vi "TurnToAngle-C.vi"(11 "Params":string[][](array[string])) -> ()   [LabVIEW 2017]
uses:
  C:/Users/Bendethic/Documents/LabVIEW Data/Projects/2018 Power Up/FRC_PracticeBot-2018/Robot Project/Framework/Robot Global Data.vi
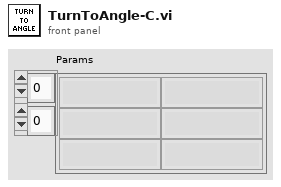
[diagram p1: front panel]
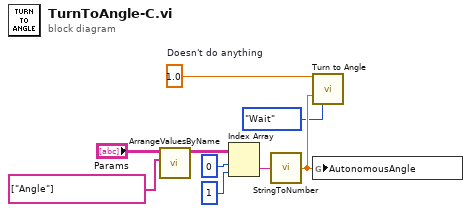
[diagram p0: block diagram]
diagram:
  w7 = 1.0  # Doesn't do anything
  n1 = call "ArrangeValuesByName.vi"("Names"=string[] ["Angle"], "Names/Values in"="Params") -> ("Names/Values Out"=w5:string[][])  [unwired: 9 in]
  n2 = Index Array(array=w5, index (row)=0, index (col)=1) -> (element=w1:string)
  n3 = call "StringToNumber.vi"("String"=w1) -> ("Output"=w9:dbl)
  n4 = call "Turn to Angle.vi"("Speed"=w7, "Target Angle"=w9, "Synchronication"=enum16{"Start", "Wait"}."Wait") -> ()  [unwired: 12 in, 1 out]
  n5 = global write "Robot Global Data.vi" "AutonomousAngle"(w9) -> ()
